vi "Boolean Latch.vi"(11 "Button Pushed?":bool) -> (2 "Toggle Button":bool, 3 "Hot Button":bool)   [LabVIEW 2017]
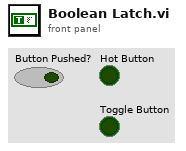
[diagram p1: front panel]
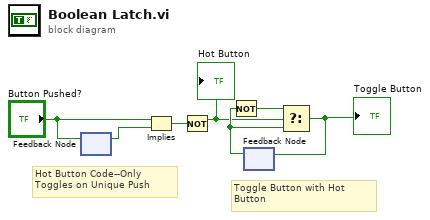
[diagram p0: block diagram]
diagram:
  # "Toggle Button with Hot Button"
  # "Hot Button Code--Only \nToggles on Unique Push"
  n1 = feedback #1() -> (w6:bool)  [unwired: 1 in]
  n2 = feedback-in #1("Button Pushed?") -> ()
  n3 = Implies(1:w6, 2:"Button Pushed?") -> (0:w1:bool)
  n4 = Not(x=w1) -> (.not. x?=w2:bool)
  "Hot Button" <- w2
  n5 = feedback #2() -> (w4:bool)  [unwired: 1 in]
  n6 = Not(x=w4) -> (.not. x?=w3:bool)
  n7 = Select(t=w3, s=w2, f=w4) -> (s? t:f=w5:bool)
  "Toggle Button" <- w5
  n8 = feedback-in #2(w5) -> ()
